vi "main.vi"() -> ()   [LabVIEW 2013]
uses:
  <vilib>/Platform/portaccess.llb/Out Port8.vi
  <vilib>/Platform/portaccess.llb/In Port8.vi
  <vilib>/Platform/portaccess.llb/Out Port32.vi
panel:
  out "-14":bool
  out "16":bool
  out "-17":bool
  out "-1":bool
  out "10":bool
  out "-11":bool
  out "12":bool
  out "13":bool
  out "15":bool
  out "2 2":bool
  out "3 2":bool
  out "4 2":bool
  out "5 2":bool
  out "6":bool
  out "7":bool
  out "8":bool
  out "9":bool
  in  "Puerto":i16(ring)=888 items=["3BC"=956, "378"=888, "278"=632]
  in  "Actualizar cada (ms)":u32=100
  in  "CONTROL":i8 format="%08b"
  out "STATUS":i8 format="%08b"
  out "ROSA":bool
  out "NARANJA":bool
  out "BLANCO":bool
  out "NEGRO":bool
  out "AZUL":bool
  out "AMARILLO":bool
  out "VERDE":bool
  out "ROJO":bool
  in  "stop":bool
  in  "Spoken Text":string
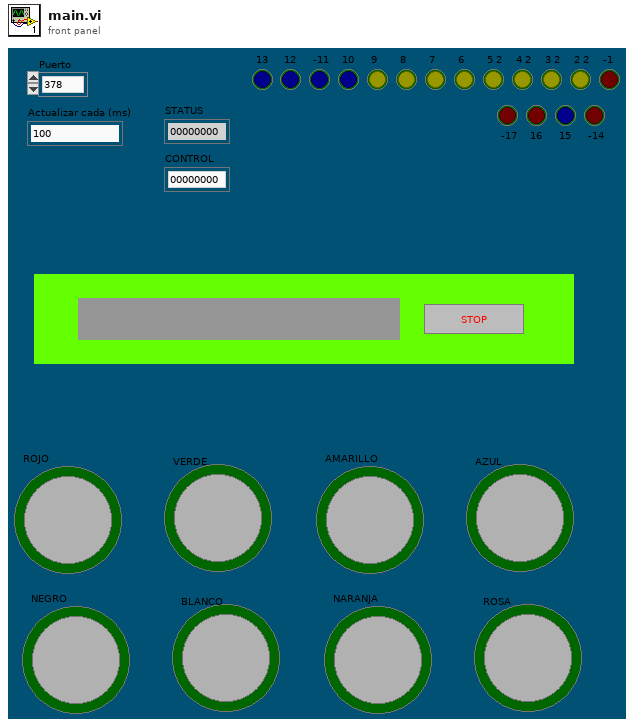
[diagram p1: front panel]
types:
  T1 = cluster{"Boolean array[0]":bool, "Boolean array[1]":bool, "Boolean array[2]":bool, "Boolean array[3]":bool, "Boolean array[4]":bool, "Boolean array[5]":bool, "Boolean array[6]":bool, "Boolean array[7]":bool, "Boolean array[8]":bool}
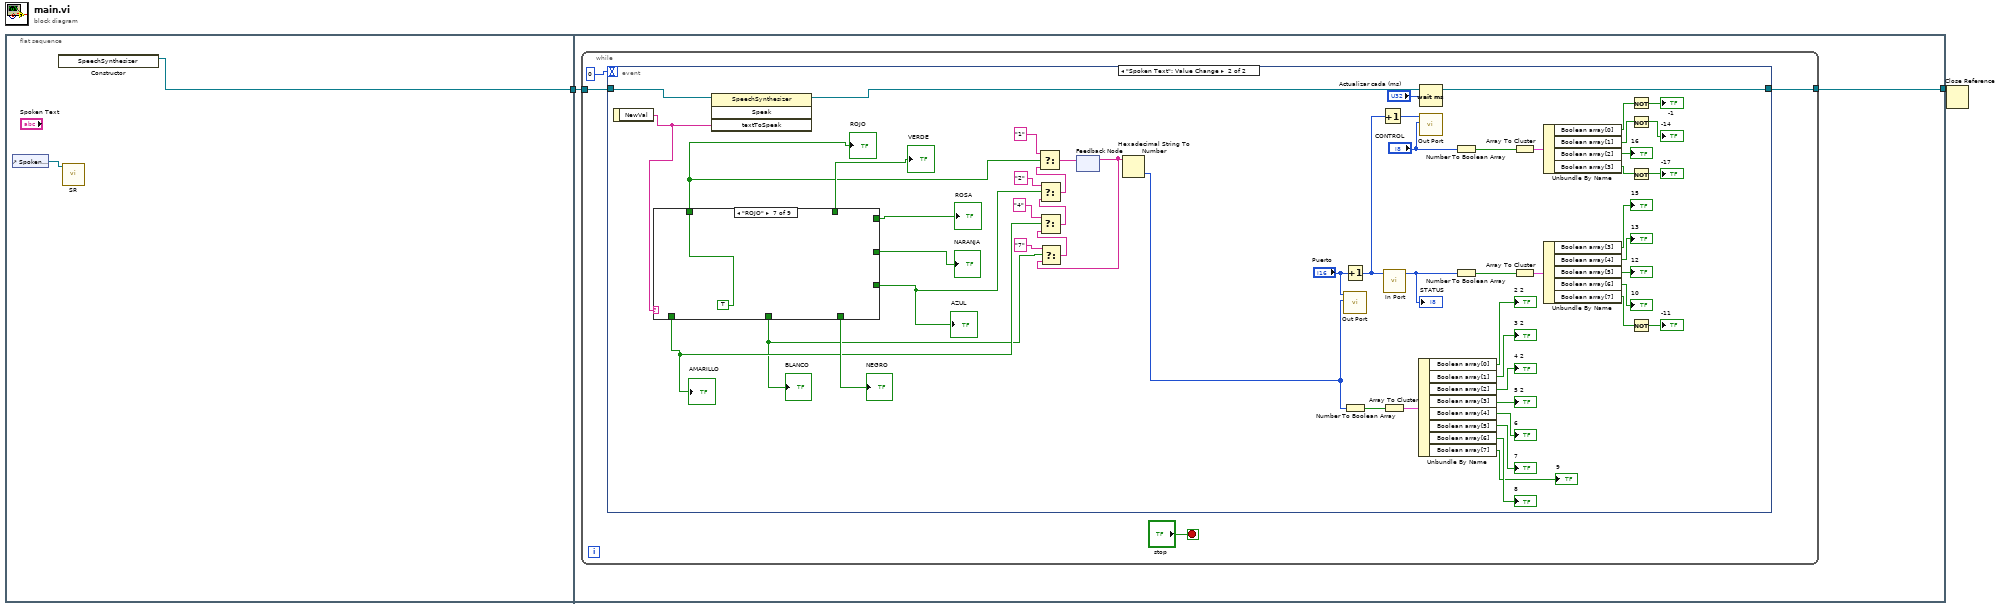
[diagram p0: block diagram]
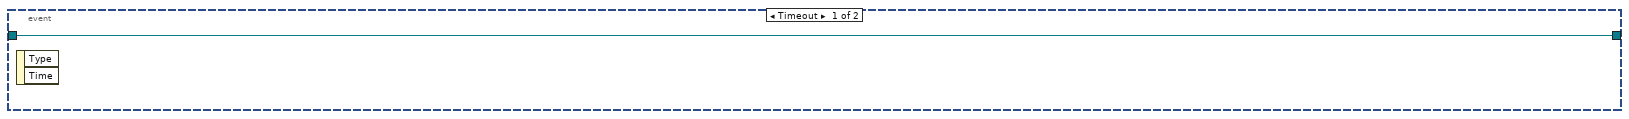
[diagram p2: hidden frame]
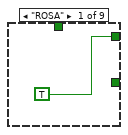
[diagram p3: hidden frame]
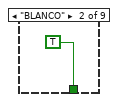
[diagram p4: hidden frame]
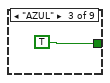
[diagram p5: hidden frame]
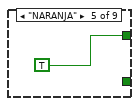
[diagram p7: hidden frame]
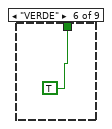
[diagram p8: hidden frame]
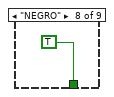
[diagram p9: hidden frame]
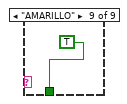
[diagram p10: hidden frame]
diagram:
  n1 = flat-sequence {
    tunnel: [w4] -> w2
    tunnel: w2 -> [w6]
    tunnel: [w5] -> w1
    frame #0 {
      n2 = control-ref of="Spoken Text"() -> (w3:refnum<vi>)
      n3 = constructor class="SpeechSynthesizer"() -> (reference out=w4:refnum<k24>)  [unwired: 3 in, 2 out]
      n4 = call "SR.vi"("Spoken text box"=w3) -> ()  [unwired: 6 in, 1 out]
    }
    frame #1 {
      n5 = while {
        tunnel: w6 -> [w9]
        tunnel: [w8] -> w5
        stop <- "stop" stop-if-true
        n6 = event shown="[1] \"Spoken Text\": Value Change" {
          selector: _ -> [_ _]
          dyn-events: _ -> [_ _]
          timeout: 0 -> [_ _]
          tunnel: w9 -> [w11 w65]
          tunnel: [w11 w64] -> w8
          event Timeout {
            n7 = event-data() -> ()  [unwired: 1 in, 2 out]
          }
          event "Spoken Text": Value Change {
            n8 = event-data() -> ("NewVal"=w62:string)  [unwired: 1 in]
            n9 = case shown="\"ROJO\"" w62 {
              tunnel: [_ _ _ _ _ _ TRUE ("Boolean") _ _] -> w15
              tunnel: [_ _ _ _ _ TRUE ("Boolean 2") _ _ _] -> w63
              tunnel: [TRUE ("ROSA") _ _ _ _ _ _ _ _] -> w61
              tunnel: [_ _ _ _ TRUE ("NARANJA") _ _ _ _] -> w60
              tunnel: [_ _ TRUE ("AZUL") _ _ _ _ _ _] -> w14
              tunnel: [_ _ _ _ _ _ _ TRUE ("NEGRO") _] -> w59
              tunnel: [_ TRUE ("BLANCO") _ _ _ _ _ _ _] -> w12
              tunnel: [_ _ _ _ _ _ _ _ TRUE ("AMARILLO")] -> w13
              frame "ROSA" {
              }
              frame "BLANCO" {
              }
              frame "AZUL" {
              }
              frame Default {
              }
              frame "NARANJA" {
              }
              frame "VERDE" {
              }
              frame "ROJO" {
              }
              frame "NEGRO" {
              }
              frame "AMARILLO" {
              }
            }
            "ROJO" <- w15
            "VERDE" <- w63
            "ROSA" <- w61
            "NARANJA" <- w60
            "AZUL" <- w14
            "AMARILLO" <- w13
            "BLANCO" <- w12
            "NEGRO" <- w59
            n10 = invoke on="Invoke Node" class="SpeechSynthesizer" method="Speak"(reference=w65, "textToSpeak"=w62) -> (reference out=w64:refnum<k24>)  [unwired: 2 in, 3 out]
            n11 = feedback #1() -> (w16:string)  [unwired: 1 in]
            n12 = Select(t="7" ("Command"), s=w12, f=w16) -> (s? t:f=w20:string)
            n13 = Select(t="4" ("Command"), s=w13, f=w20) -> (s? t:f=w22:string)
            n14 = Select(t="2" ("Command"), s=w14, f=w22) -> (s? t:f=w24:string)
            n15 = Select(t="1" ("Command"), s=w15, f=w24) -> (s? t:f=w17:string)
            n16 = feedback-in #1(w17) -> ()
            n17 = Hexadecimal String To Number(string=w16) -> (number=w18:u32)  [unwired: 2 in, 1 out]
            n18 = Increment(x="Puerto") -> (x+1=w53:i16)
            n19 = call-poly <vilib>:"Out Port.vi"("write value"=w18, "address"="Puerto") -> ()  [unwired: 1 in, 7 out]
            n20 = Number To Boolean Array(number=w18) -> (Boolean array=w52:bool[])
            n21 = Increment(x=w53) -> (x+1=w57:i16)
            n22 = Array To Cluster(array=w52) -> (cluster=w51:T1)
            n23 = call-poly <vilib>:"In Port.vi"("address"=w53) -> ("data read"=w55:i8)  [unwired: 1 in, 7 out]
            "STATUS" <- w55
            n24 = Unbundle By Name(w51) -> ("Boolean array[0]"=→"2 2":bool, "Boolean array[1]"=→"3 2":bool, "Boolean array[2]"=→"4 2":bool, "Boolean array[3]"=→"5 2":bool, "Boolean array[4]"=→"6":bool, "Boolean array[5]"=→"7":bool, "Boolean array[6]"=→"8":bool, "Boolean array[7]"=→"9":bool)
            n25 = Wait (ms)(milliseconds to wait="Actualizar cada (ms)") -> ()  [unwired: 1 out]
            n26 = call-poly <vilib>:"Out Port.vi"("write value"="CONTROL", "address"=w57) -> ()  [unwired: 1 in, 7 out]
            n27 = Number To Boolean Array(number="CONTROL") -> (Boolean array=w47:bool[])
            n28 = Number To Boolean Array(number=w55) -> (Boolean array=w49:bool[])
            n29 = Array To Cluster(array=w47) -> (cluster=w48:T1)
            n30 = Array To Cluster(array=w49) -> (cluster=w50:T1)
            n31 = Unbundle By Name(w48) -> ("Boolean array[0]"=w27:bool, "Boolean array[1]"=w29:bool, "Boolean array[2]"=→"16":bool, "Boolean array[3]"=w31:bool)
            n32 = Unbundle By Name(w50) -> ("Boolean array[3]"=→"15":bool, "Boolean array[4]"=→"13":bool, "Boolean array[5]"=→"12":bool, "Boolean array[6]"=→"10":bool, "Boolean array[7]"=w33:bool)
            n33 = Not(x=w27) -> (.not. x?=→"-1":bool)
            n34 = Not(x=w29) -> (.not. x?=→"-14":bool)
            n35 = Not(x=w31) -> (.not. x?=→"-17":bool)
            n36 = Not(x=w33) -> (.not. x?=→"-11":bool)
          }
        }
      }
    }
  }
  n37 = Close Reference(reference=w1) -> ()  [unwired: 1 in, 1 out]
